vi "qpsk using bpsk.vi"() -> ()   [LabVIEW 2014]
panel:
  out "carrier 1":dynamicdata(graph) caption="Sine"
  out "carrier 2":dynamicdata(graph) caption="Sine"
  out "Square message singal 2":dynamicdata(graph) caption="Square"
  out "Square message signal1":dynamicdata(graph) caption="Square"
  out "QPSK graph":dynamicdata(graph)
  out "bpsk 2":dynamicdata(graph)
  out "bpsk 1":dynamicdata(graph)
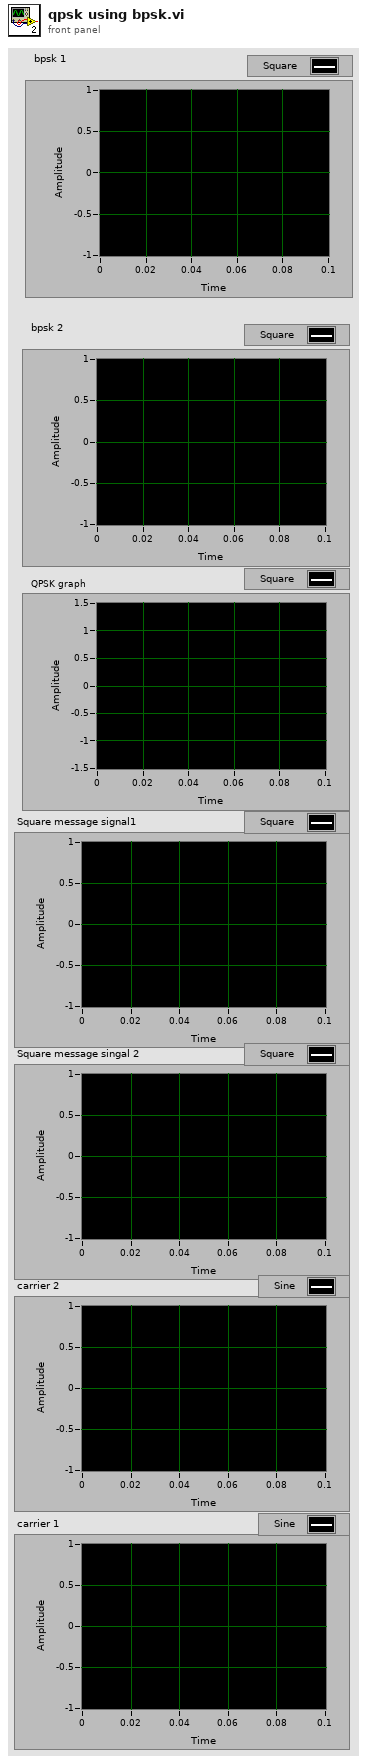
[diagram p1: front panel]
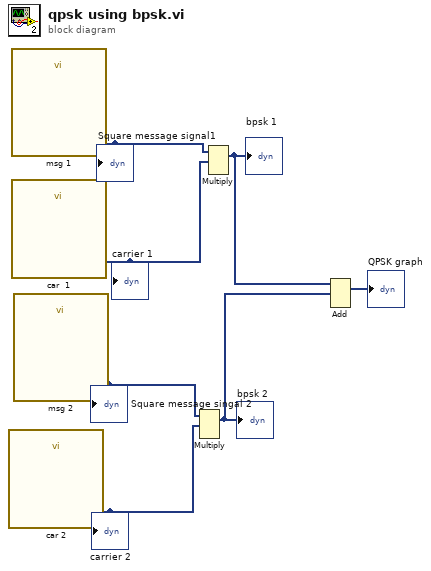
[diagram p0: block diagram]
diagram:
  n1 = call "car 2"() -> ("Sine"=w4:dynamicdata)  [unwired: 14 in, 1 out]
  "carrier 2" <- w4
  n2 = call "msg 1"() -> ("Square"=w7:dynamicdata)  [unwired: 14 in, 1 out]
  "Square message signal1" <- w7
  n3 = call "car  1"() -> ("Sine"=w6:dynamicdata)  [unwired: 14 in, 1 out]
  "carrier 1" <- w6
  n4 = call "msg 2"() -> ("Square"=w5:dynamicdata)  [unwired: 14 in, 1 out]
  "Square message singal 2" <- w5
  n5 = Multiply(1:w4, 2:w5) -> (0:w2:dynamicdata)  [unwired: 1 in, 1 out]
  "bpsk 2" <- w2
  n6 = Multiply(1:w6, 2:w7) -> (0:w3:dynamicdata)  [unwired: 1 in, 1 out]
  "bpsk 1" <- w3
  n7 = Add(1:w2, 2:w3) -> (0:→"QPSK graph":dynamicdata)  [unwired: 1 in, 1 out]
